vi "FilePath_raw_signal_temperature.vi"(0 "base folder path":path=path "F:/disk E/OOK/NI_Data") -> (1 "Raw_data_path":path)   [LabVIEW 2014]
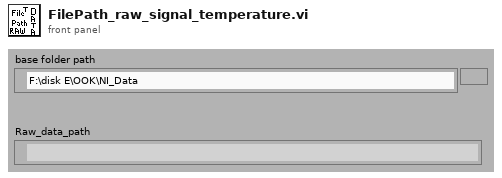
[diagram p1: front panel]
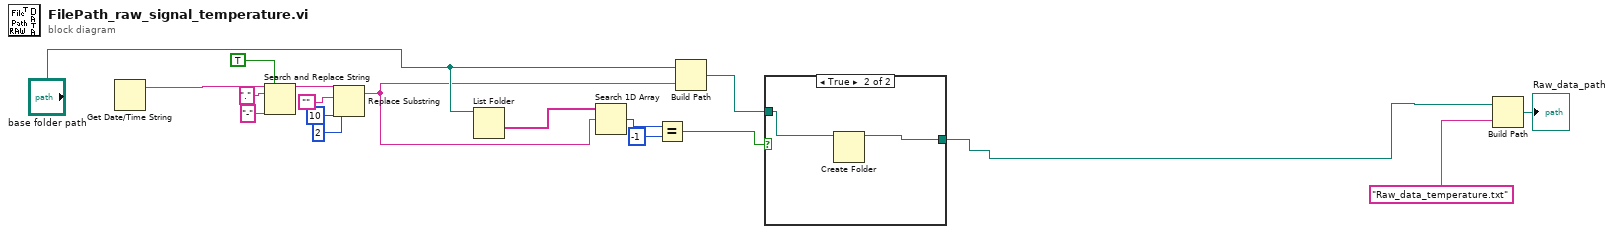
[diagram p0: block diagram]
diagram:
  n1 = Get Date/Time String() -> (date string=w18:string)  [unwired: 3 in, 1 out]
  n2 = Search and Replace String(replace all?=TRUE ("replace all? (F)"), input string=w18, search string=".", replace string="-" ("replace string (\"\")")) -> (result string=w5:string)  [unwired: 4 in, 3 out]
  n3 = Replace Substring(2:2 ("length (len. of substring)"), 3:10 ("offset (0)"), 4:"", 5:w5) -> (1:w6:string)  [unwired: 1 out]
  n4 = List Folder(path="base folder path") -> (folder names=w13:string[])  [unwired: 3 in, 3 out]
  n5 = Search 1D Array(1D array=w13, element=w6) -> (index of element=w12:i32)  [unwired: 1 in]
  n6 = Equal?(x=w12, y=-1) -> (x = y?=w10:bool)
  n7 = Build Path(base path="base folder path", name or relative path=w6) -> (appended path=w9:path)
  n8 = case shown="True" w10 {
    tunnel: w9 -> [w19 w21]
    tunnel: [w19 w20] -> w1
    frame False {
    }
    frame True {
      n9 = Create Folder(path (use dialog)=w21) -> (created path=w20:path)  [unwired: 2 in, 2 out]
    }
  }
  n10 = Build Path(base path=w1, name or relative path="Raw_data_temperature.txt") -> (appended path=→"Raw_data_path":path)
